vi "lcd_display.vi"() -> ()   [LabVIEW 2015]
panel:
  in  "background":string
  in  "char_color":string
  in  "String":string
  in  "y":dbl
  in  "x":dbl
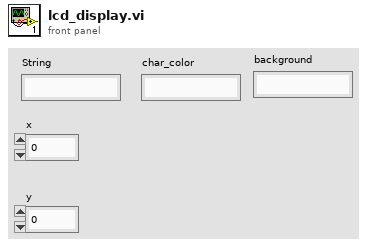
[diagram p1: front panel]
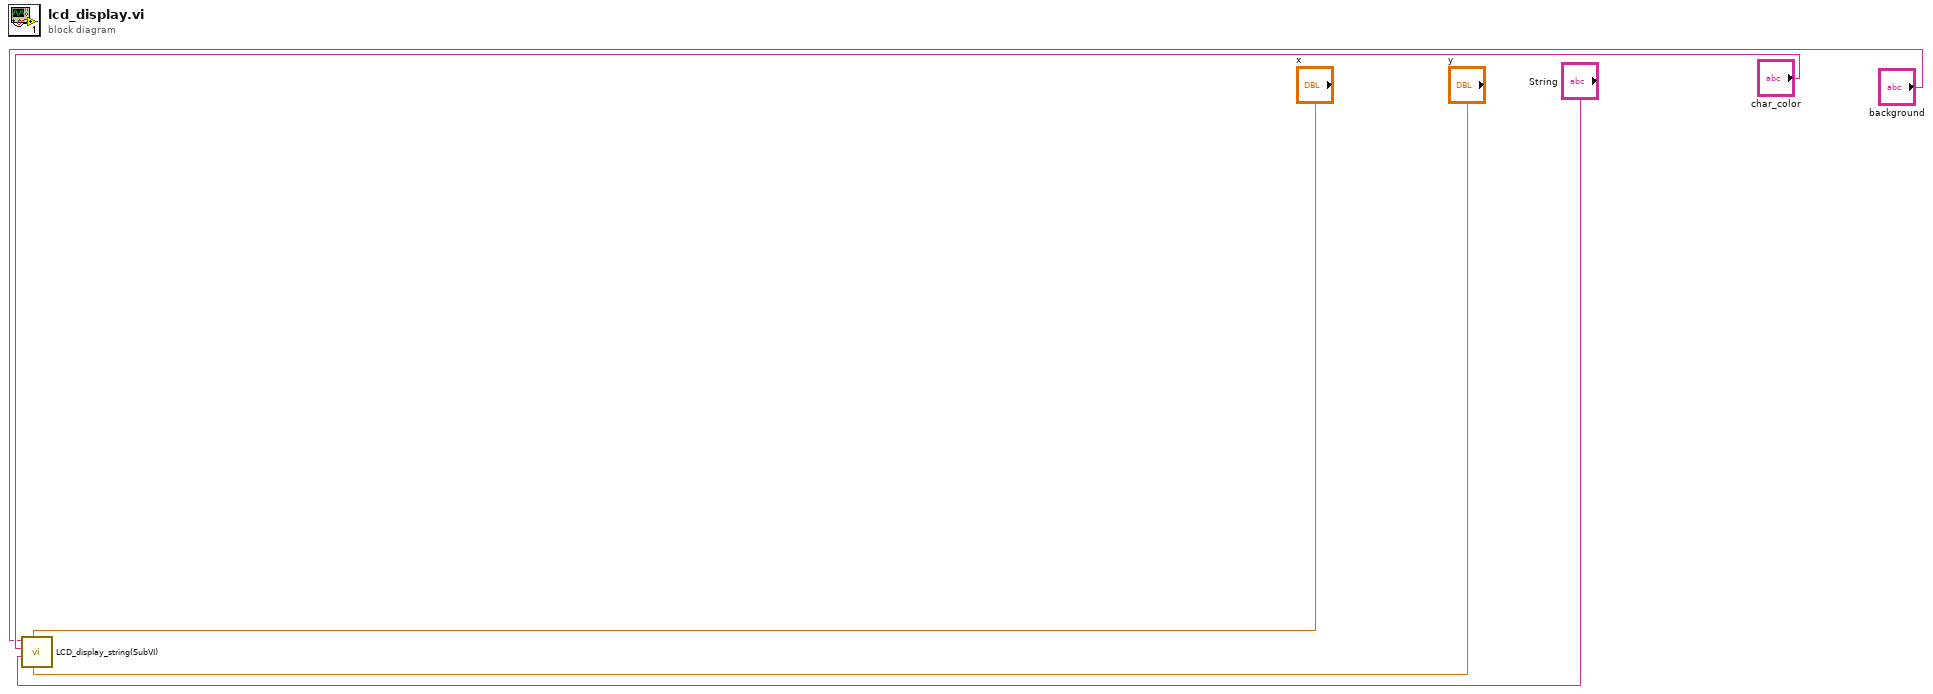
[diagram p0: block diagram]
diagram:
  n1 = call "LCD_display_string(SubVI).vi"("y"="y", "x"="x", "String"="String", "char_color"="char_color", "background"="background") -> ()  [unwired: 7 in]
